vi "PBI_MFA_Interface_IACT_InitialSetup1_DefaultFactory.vi"(9 "Meas Curr":bool, 11 "FacDefault":bool) -> (1 "CurrentMeas2_at5V":sgl, 2 "CurrentMeas1_at5V":sgl, 3 "FactoryDefaultError":bool)   [LabVIEW 2011]
panel:
  out "error CurrentMeas2_at5V":errorcluster
  out "error CurrentMeas1_at5V":errorcluster
  out "error FactoryDefaults":errorcluster
  out "AAABuild":i32
  in  "MintController":refnum<k7>(container)
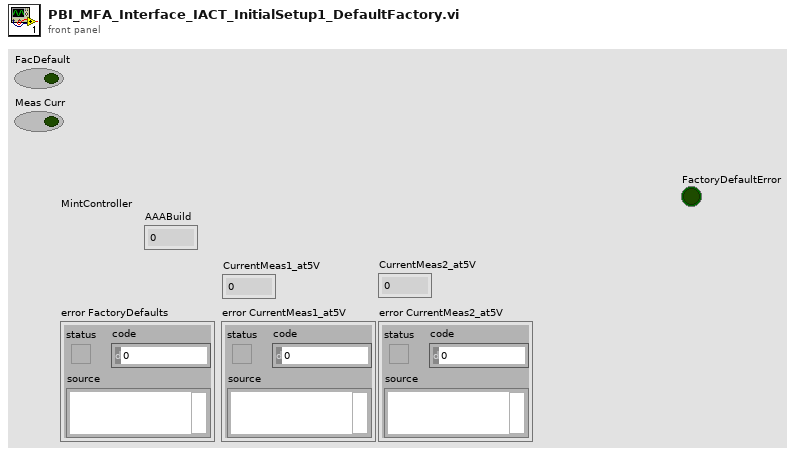
[diagram p1: front panel]
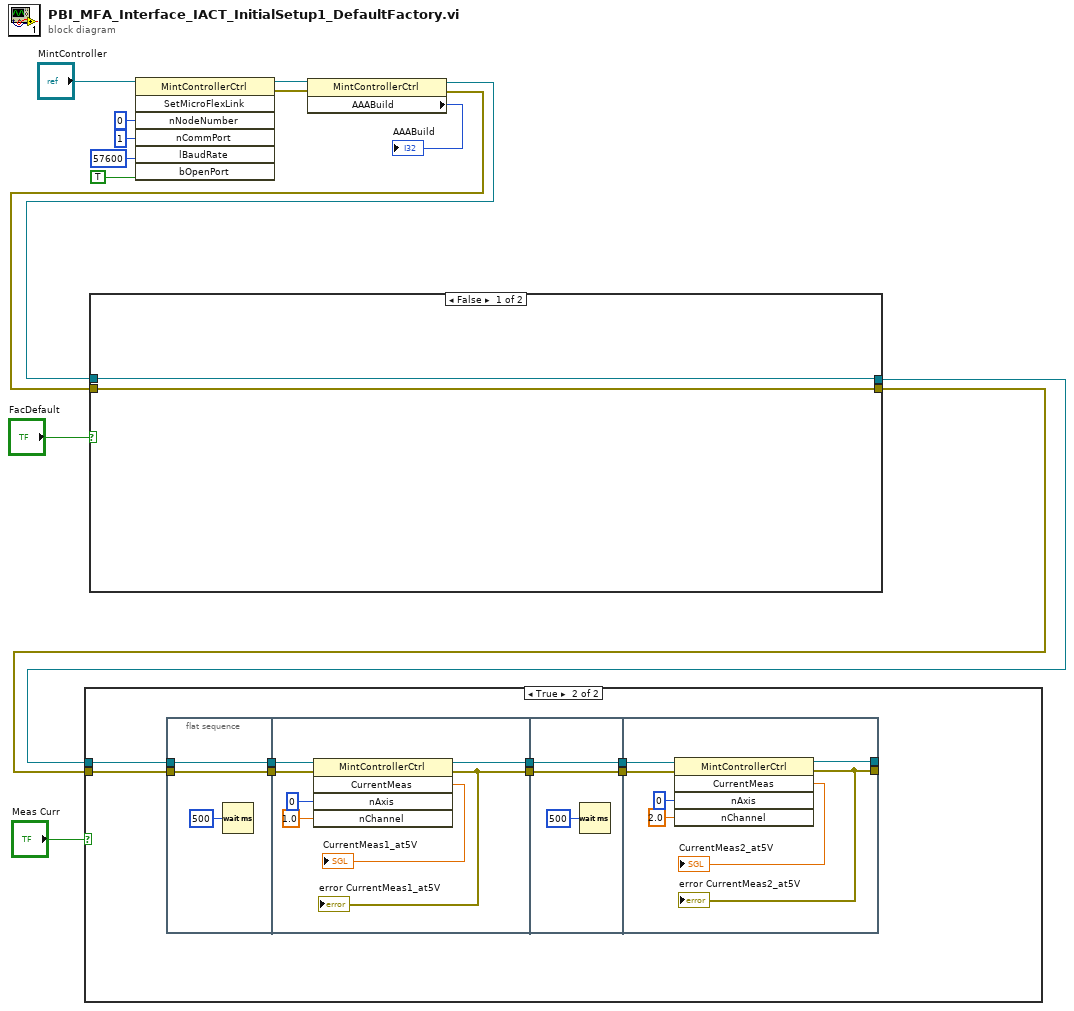
[diagram p0: block diagram]
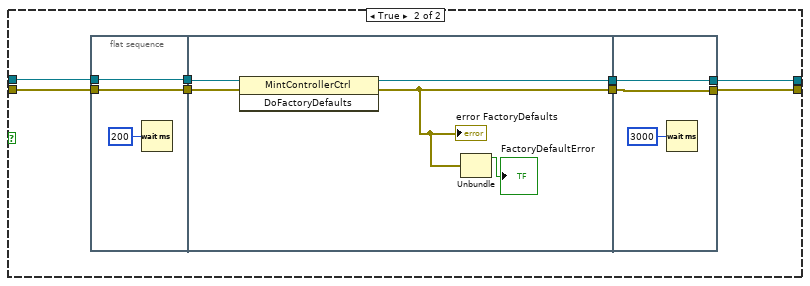
[diagram p2: hidden frame]
diagram:
  n1 = invoke class="MintControllerCtrl" method="SetMicroFlexLink"(reference="MintController", "nNodeNumber"=i16 0, "nCommPort"=i16 1, "lBaudRate"=57600, "bOpenPort"=TRUE) -> (reference out=w14:refnum<k7>, error out=w8:errorcluster)  [unwired: 2 in, 5 out]
  n2 = property class="MintControllerCtrl"(reference=w14, error in=w8) -> (reference out=w5:refnum<k7>, error out=w6:errorcluster, "AAABuild"=→"AAABuild":i32)
  n3 = case shown="False" "FacDefault" {
    tunnel: w6 -> [w15 w20]
    tunnel: w5 -> [w16 w19]
    tunnel: [w16 w18] -> w4
    tunnel: [w15 w17] -> w3
    frame False {
    }
    frame True {
      n4 = flat-sequence {
        tunnel: [w27] -> w24
        tunnel: [w26] -> w23
        tunnel: w20 -> [w27]
        tunnel: w19 -> [w26]
        tunnel: w24 -> [w32]
        tunnel: w23 -> [w31]
        tunnel: [w29] -> w22
        tunnel: [w30] -> w21
        tunnel: w22 -> [w33]
        tunnel: w21 -> [w34]
        tunnel: [w34] -> w18
        tunnel: [w33] -> w17
        frame #0 {
          n5 = Wait (ms)(milliseconds to wait=u32 200) -> ()  [unwired: 1 out]
        }
        frame #1 {
          n6 = invoke class="MintControllerCtrl" method="DoFactoryDefaults"(reference=w31, error in=w32) -> (reference out=w30:refnum<k7>, error out=w29:errorcluster)  [unwired: 1 in, 1 out]
          "error FactoryDefaults" <- w29
          n7 = Unbundle(w29) -> ("status"=→"FactoryDefaultError":bool)  [unwired: 2 out]
        }
        frame #2 {
          n8 = Wait (ms)(milliseconds to wait=u32 3000) -> ()  [unwired: 1 out]
        }
      }
    }
  }
  n9 = case shown="True" "Meas Curr" {
    tunnel: w4 -> [_ w37]
    tunnel: w3 -> [_ w36]
    frame False {
    }
    frame True {
      n10 = flat-sequence {
        tunnel: [w45] -> w43
        tunnel: [w44] -> w42
        tunnel: w37 -> [w45]
        tunnel: w36 -> [w44]
        tunnel: w43 -> [w53]
        tunnel: [w50] -> w41
        tunnel: [w49] -> w40
        tunnel: w42 -> [w47]
        tunnel: w41 -> [w55]
        tunnel: w40 -> [w54]
        tunnel: [w55] -> w39
        tunnel: [w54] -> w38
        tunnel: w39 -> [w62]
        tunnel: w38 -> [w63]
        tunnel: [w60] -> _
        tunnel: [w59] -> _
        frame #0 {
          n11 = Wait (ms)(milliseconds to wait=u32 500) -> ()  [unwired: 1 out]
        }
        frame #1 {
          n12 = invoke class="MintControllerCtrl" method="CurrentMeas"(reference=w53, error in=w47, "nAxis"=i16 0 ("nParam"), "nChannel"=sgl 1.0 ("newValue")) -> (reference out=w49:refnum<k7>, error out=w50:errorcluster, "CurrentMeas"=→"CurrentMeas1_at5V":sgl)  [unwired: 1 in, 2 out]
          "error CurrentMeas1_at5V" <- w50
        }
        frame #2 {
          n13 = Wait (ms)(milliseconds to wait=u32 500) -> ()  [unwired: 1 out]
        }
        frame #3 {
          n14 = invoke class="MintControllerCtrl" method="CurrentMeas"(reference=w63, error in=w62, "nAxis"=i16 0, "nChannel"=sgl 2.0 ("newValue")) -> (reference out=w59:refnum<k7>, error out=w60:errorcluster, "CurrentMeas"=→"CurrentMeas2_at5V":sgl)  [unwired: 1 in, 2 out]
          "error CurrentMeas2_at5V" <- w60
        }
      }
    }
  }
